vi "create.Messages.from.Variants.vi"(11 "Messages.Variant":variant[](array[variant])) -> (3 "Messages":refnum<class "MessageBase.lvclass">[](array[class]))   [LabVIEW 2020]
uses:
  MessageBase/MessageBase.lvclass
  Time/Time.Parameters.ctl
  AddOrder/AddOrderLong.Parameters.ctl
  AddOrder/AddOrderShort.Parameters.ctl
  AddOrder/AddOrderExpanded.Parameters.ctl
  OrderExecuted/OrderExecuted.Parameters.ctl
  OrderExecuted/OrderExecutedAtPriceSize.Parameters.ctl
  ReduceSize/ReduceSizeLong.Parameters.ctl
  ReduceSize/ReduceSizeShort.Parameters.ctl
  ModifyOrder/ModifyOrderLong.Parameters.ctl
  ModifyOrder/ModifyOrderShort.Parameters.ctl
  DeleteOrder/DeleteOrder.Parameters.ctl
  Trade/TradeLong.Parameters.ctl
  Trade/TradeShort.Parameters.ctl
  Trade/TradeExpanded.Parameters.ctl
  AddOrder/AddOrderShort.lvclass
  C:/work/fpganow/Market.Data.PoC/submodules/Market.Data.Bats.Parser/host/pitch/MessageBase/MessageBase.lvclass
  AddOrder/AddOrderExpanded.lvclass
  OrderExecuted/OrderExecuted.lvclass
  OrderExecuted/OrderExecutedAtPriceSize.lvclass
  ReduceSize/ReduceSizeLong.lvclass
  ReduceSize/ReduceSizeShort.lvclass
  ModifyOrder/ModifyOrderLong.lvclass
  ModifyOrder/ModifyOrderShort.lvclass
  DeleteOrder/DeleteOrder.lvclass
  Trade/TradeLong.lvclass
  Trade/TradeShort.lvclass
  Trade/TradeExpanded.lvclass
  <vilib>/Utility/Data Type/NI_Data Type.lvlib
  Time/Time.lvclass
  AddOrder/AddOrderLong.lvclass
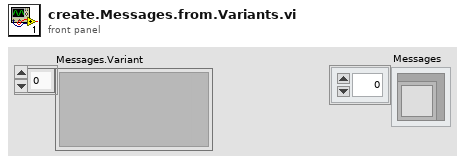
[diagram p1: front panel]
types:
  T1 = typedef "Time.lvclass/Time.Parameters.ctl" = cluster{"Time":u32}
  T2 = typedef "AddOrderLong.lvclass/AddOrderLong.Parameters.ctl" = cluster{"Time Offset":u32, "Order Id":string, "Quantity":u32, "Symbol":string, "Side Indicator":string, "Price":dbl}
  T3 = typedef "AddOrderShort.lvclass/AddOrderShort.Parameters.ctl" = cluster{"Time Offset":u32, "Order Id":string, "Quantity":u32, "Symbol":string, "Side Indicator":string, "Price":dbl}
  T4 = typedef "AddOrderExpanded.lvclass/AddOrderExpanded.Parameters.ctl" = cluster{"Time Offset":u32, "Order Id":string, "Quantity":u32, "Symbol":string, "Side Indicator":string, "Price":dbl, "Participant Id":string, "Customer Indicator":string}
  T5 = typedef "OrderExecuted.lvclass/OrderExecuted.Parameters.ctl" = cluster{"Time Offset":u32, "Order Id":string, "Executed Quantity":u32, "Execution Id":string}
  T6 = typedef "OrderExecutedAtPriceSize.lvclass/OrderExecutedAtPriceSize.Parameters.ctl" = cluster{"Time Offset":u32, "Order Id":string, "Executed Quantity":u32, "Execution Id":string, "Remaining Quantity":u32, "Price":dbl}
  T7 = typedef "ReduceSizeLong.lvclass/ReduceSizeLong.Parameters.ctl" = cluster{"Time Offset":u32, "Order Id":string, "Canceled Quantity":u32}
  T8 = typedef "ReduceSizeShort.lvclass/ReduceSizeShort.Parameters.ctl" = cluster{"Time Offset":u32, "Order Id":string, "Canceled Quantity":u16}
  T9 = typedef "ModifyOrderLong.lvclass/ModifyOrderLong.Parameters.ctl" = cluster{"Time Offset":u32, "Order Id":string, "Quantity":u32, "Price":dbl, "Modify Flags":u8}
  T10 = typedef "ModifyOrderShort.lvclass/ModifyOrderShort.Parameters.ctl" = cluster{"Time Offset":u32, "Order Id":string, "Quantity":u32, "Price":u16, "Modify Flags":u8}
  T11 = typedef "DeleteOrder.lvclass/DeleteOrder.Parameters.ctl" = cluster{"Time Offset":u32, "Order Id":string}
  T12 = typedef "TradeLong.lvclass/TradeLong.Parameters.ctl" = cluster{"Time Offset":u32, "Order Id":string, "Execution Id":string, "Quantity":u32, "Price":dbl, "Side Indicator":string, "Symbol":string}
  T13 = typedef "TradeShort.lvclass/TradeShort.Parameters.ctl" = cluster{"Time Offset":u32, "Order Id":string, "Execution Id":string, "Quantity":u32, "Price":dbl, "Side Indicator":string, "Symbol":string}
  T14 = typedef "TradeExpanded.lvclass/TradeExpanded.Parameters.ctl" = cluster{"Time Offset":u32, "Order Id":string, "Side Indicator":string, "Quantity":u32, "Symbol":string, "Price":dbl, "Execution Id":string}
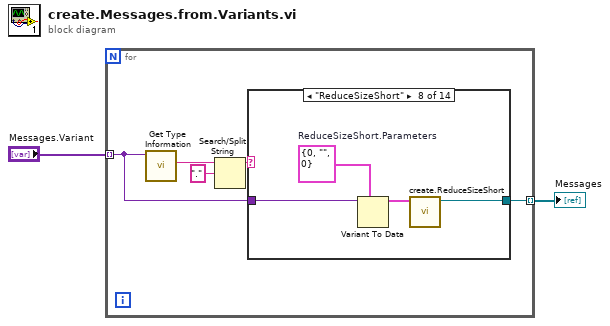
[diagram p0: block diagram]
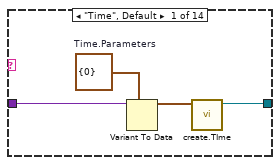
[diagram p2: hidden frame]
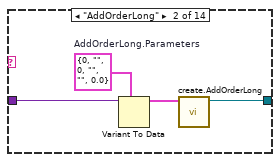
[diagram p3: hidden frame]
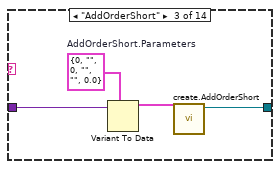
[diagram p4: hidden frame]
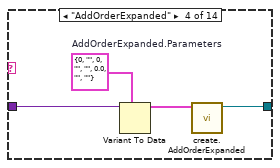
[diagram p5: hidden frame]
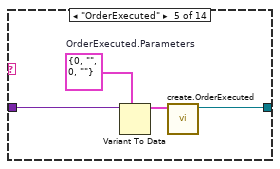
[diagram p6: hidden frame]
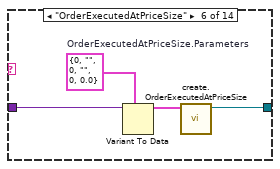
[diagram p7: hidden frame]
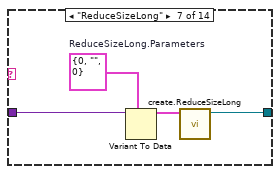
[diagram p8: hidden frame]
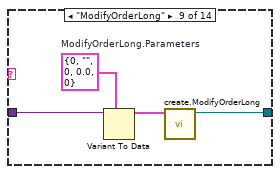
[diagram p9: hidden frame]
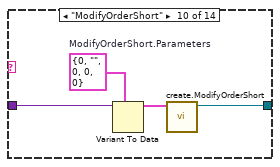
[diagram p10: hidden frame]
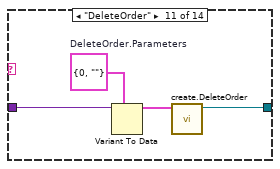
[diagram p11: hidden frame]
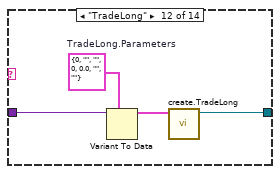
[diagram p12: hidden frame]
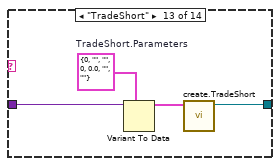
[diagram p13: hidden frame]
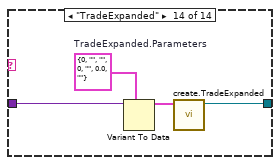
[diagram p14: hidden frame]
diagram:
  n1 = for {
    tunnel: "Messages.Variant" -> [w7] mode=indexing
    tunnel: [w6] -> w1 mode=indexing
    n2 = call <vilib>:"Get Type Information.vi"("variant"=w7) -> ("name"=w5:string)  [unwired: 6 in, 4 out]
    n3 = Search/Split String(string=w5, search string/char (-)=".") -> (substring before match=w3:string)  [unwired: 1 in, 2 out]
    n4 = case shown="\"ReduceSizeShort\"" w3 {
      tunnel: [w11 w15 w19 w23 w27 w31 w35 w39 w43 w47 w51 w55 w59 w63] -> w6
      tunnel: w7 -> [w9 w14 w17 w22 w26 w30 w34 w38 w42 w46 w50 w54 w58 w62]
      frame "Time", Default {
        w10 = T1 {"Time"=0}  # Time.Parameters
        n5 = Variant To Data(type=w10, Variant=w9) -> (data=w8:T1)  [unwired: 1 in, 1 out]
        n6 = call "create.TIme.vi"("Time.Parameters"=w8) -> ("MessageBase out"=w11:refnum<class "MessageBase.lvclass">)  [unwired: 8 in, 2 out]
      }
      frame "AddOrderLong" {
        w13 = T2 {"Time Offset"=0, "Order Id"="", "Quantity"=0, "Symbol"="", "Side Indicator"="", "Price"=0.0}  # AddOrderLong.Parameters
        n7 = Variant To Data(type=w13, Variant=w14) -> (data=w12:T2)  [unwired: 1 in, 1 out]
        n8 = call "create.AddOrderLong.vi"("AddOrderLong.Parameters"=w12) -> ("MessageBase out"=w15:refnum<class "MessageBase.lvclass">)  [unwired: 9 in, 1 out]
      }
      frame "AddOrderShort" {
        w18 = T3 {"Time Offset"=0, "Order Id"="", "Quantity"=0, "Symbol"="", "Side Indicator"="", "Price"=0.0}  # AddOrderShort.Parameters
        n9 = Variant To Data(type=w18, Variant=w17) -> (data=w16:T3)  [unwired: 1 in, 1 out]
        n10 = call "create.AddOrderShort.vi"("AddOrderShort.Parameters"=w16) -> ("MessageBase out"=w19:refnum<class "AddOrderShort.lvclass">)  [unwired: 9 in, 1 out]
      }
      frame "AddOrderExpanded" {
        w21 = T4 {"Time Offset"=0, "Order Id"="", "Quantity"=0, "Symbol"="", "Side Indicator"="", "Price"=0.0, "Participant Id"="", "Customer Indicator"=""}  # AddOrderExpanded.Parameters
        n11 = Variant To Data(type=w21, Variant=w22) -> (data=w20:T4)  [unwired: 1 in, 1 out]
        n12 = call "create.AddOrderExpanded.vi"("AddOrderExpanded.Parameters"=w20) -> ("MessageBase out"=w23:refnum<class "AddOrderExpanded.lvclass">)  [unwired: 9 in, 1 out]
      }
      frame "OrderExecuted" {
        w25 = T5 {"Time Offset"=0, "Order Id"="", "Executed Quantity"=0, "Execution Id"=""}  # OrderExecuted.Parameters
        n13 = Variant To Data(type=w25, Variant=w26) -> (data=w24:T5)  [unwired: 1 in, 1 out]
        n14 = call "create.OrderExecuted.vi"("OrderExecuted.Parameters"=w24) -> ("MessageBase out"=w27:refnum<class "OrderExecuted.lvclass">)  [unwired: 9 in, 1 out]
      }
      frame "OrderExecutedAtPriceSize" {
        w29 = T6 {"Time Offset"=0, "Order Id"="", "Executed Quantity"=0, "Execution Id"="", "Remaining Quantity"=0, "Price"=0.0}  # OrderExecutedAtPriceSize.Parameters
        n15 = Variant To Data(type=w29, Variant=w30) -> (data=w28:T6)  [unwired: 1 in, 1 out]
        n16 = call "create.OrderExecutedAtPriceSize.vi"("OrderExecutedAtPriceSize.Parameters"=w28) -> ("MessageBase out"=w31:refnum<class "OrderExecutedAtPriceSize.lvclass">)  [unwired: 9 in, 1 out]
      }
      frame "ReduceSizeLong" {
        w33 = T7 {"Time Offset"=0, "Order Id"="", "Canceled Quantity"=0}  # ReduceSizeLong.Parameters
        n17 = Variant To Data(type=w33, Variant=w34) -> (data=w32:T7)  [unwired: 1 in, 1 out]
        n18 = call "create.ReduceSizeLong.vi"("ReduceSizeLong.Parameters"=w32) -> ("ReduceSizeLong"=w35:refnum<class "ReduceSizeLong.lvclass">)  [unwired: 8 in, 2 out]
      }
      frame "ReduceSizeShort" {
        w37 = T8 {"Time Offset"=0, "Order Id"="", "Canceled Quantity"=0}  # ReduceSizeShort.Parameters
        n19 = Variant To Data(type=w37, Variant=w38) -> (data=w36:T8)  [unwired: 1 in, 1 out]
        n20 = call "create.ReduceSizeShort.vi"("ReduceSizeShort.Parameters"=w36) -> ("MessageBase out"=w39:refnum<class "ReduceSizeShort.lvclass">)  [unwired: 8 in, 2 out]
      }
      frame "ModifyOrderLong" {
        w41 = T9 {"Time Offset"=0, "Order Id"="", "Quantity"=0, "Price"=0.0, "Modify Flags"=0}  # ModifyOrderLong.Parameters
        n21 = Variant To Data(type=w41, Variant=w42) -> (data=w40:T9)  [unwired: 1 in, 1 out]
        n22 = call "create.ModifyOrderLong.vi"("ModifyOrderLong.Parameters"=w40) -> ("MessageBase out"=w43:refnum<class "ModifyOrderLong.lvclass">)  [unwired: 8 in, 2 out]
      }
      frame "ModifyOrderShort" {
        w45 = T10 {"Time Offset"=0, "Order Id"="", "Quantity"=0, "Price"=0, "Modify Flags"=0}  # ModifyOrderShort.Parameters
        n23 = Variant To Data(type=w45, Variant=w46) -> (data=w44:T10)  [unwired: 1 in, 1 out]
        n24 = call "create.ModifyOrderShort.vi"("ModifyOrderShort.Parameters"=w44) -> ("MessageBase out"=w47:refnum<class "ModifyOrderShort.lvclass">)  [unwired: 8 in, 2 out]
      }
      frame "DeleteOrder" {
        w49 = T11 {"Time Offset"=0, "Order Id"=""}  # DeleteOrder.Parameters
        n25 = Variant To Data(type=w49, Variant=w50) -> (data=w48:T11)  [unwired: 1 in, 1 out]
        n26 = call "create.DeleteOrder.vi"("DeleteOrder.Parameters"=w48) -> ("MessageBase out"=w51:refnum<class "DeleteOrder.lvclass">)  [unwired: 8 in, 2 out]
      }
      frame "TradeLong" {
        w53 = T12 {"Time Offset"=0, "Order Id"="", "Execution Id"="", "Quantity"=0, "Price"=0.0, "Side Indicator"="", "Symbol"=""}  # TradeLong.Parameters
        n27 = Variant To Data(type=w53, Variant=w54) -> (data=w52:T12)  [unwired: 1 in, 1 out]
        n28 = call "create.TradeLong.vi"("TradeLong.Parms"=w52) -> ("MessageBase out"=w55:refnum<class "TradeLong.lvclass">)  [unwired: 8 in, 2 out]
      }
      frame "TradeShort" {
        w57 = T13 {"Time Offset"=0, "Order Id"="", "Execution Id"="", "Quantity"=0, "Price"=0.0, "Side Indicator"="", "Symbol"=""}  # TradeShort.Parameters
        n29 = Variant To Data(type=w57, Variant=w58) -> (data=w56:T13)  [unwired: 1 in, 1 out]
        n30 = call "create.TradeShort.vi"("TradeShort.Parmeters"=w56) -> ("MessageBase out"=w59:refnum<class "TradeShort.lvclass">)  [unwired: 8 in, 2 out]
      }
      frame "TradeExpanded" {
        w61 = T14 {"Time Offset"=0, "Order Id"="", "Side Indicator"="", "Quantity"=0, "Symbol"="", "Price"=0.0, "Execution Id"=""}  # TradeExpanded.Parameters
        n31 = Variant To Data(type=w61, Variant=w62) -> (data=w60:T14)  [unwired: 1 in, 1 out]
        n32 = call "create.TradeExpanded.vi"("TradeExpanded.Parmeters"=w60) -> ("MessageBase out"=w63:refnum<class "TradeExpanded.lvclass">)  [unwired: 8 in, 2 out]
      }
    }
  }
  "Messages" <- w1
